vi "Get 2D String.vi"(5 "format string (%s)":string="%s", 7 "key description":string, 8 "sections":string[](array[string]), 9 "string":string[][](array[string]), 11 "info data":string) -> (0 "sections out":string[](array[string]), 2 "value":string[][](array[string]), 3 "info data out":string)   [LabVIEW 2019, in "infolib.lvlib"]
doc: "Reads matrix of strings. If section is entered it searches the key in the section(s)."
uses:
  infolib.lvlib
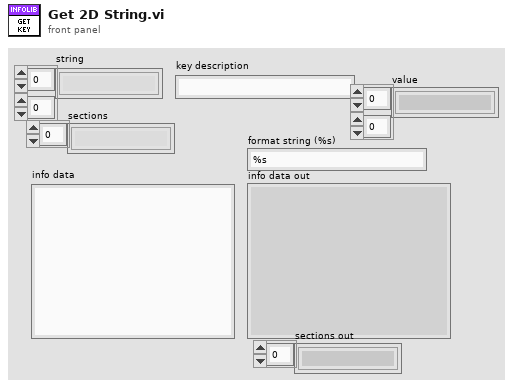
[diagram p1: front panel]
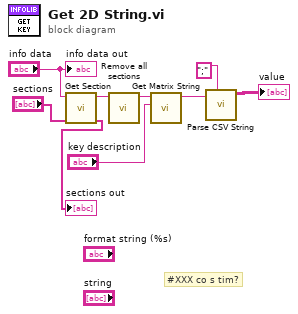
[diagram p0: block diagram]
diagram:
  # "#XXX co s tim?"
  n1 = call "Get Section.vi"("sections"="sections", "info data"="info data") -> ("sections out"=→"sections out":string[], "section part"=w9:string)  [unwired: 7 in, 1 out]
  n2 = call "Remove all sections.vi"("info data"=w9) -> ("info data out"=w7:string)  [unwired: 10 in]
  n3 = call "Get Matrix String.vi"("matrix key"="key description", "info data"=w7) -> ("matrix part"=w5:string)  [unwired: 8 in, 1 out]
  n4 = call "Parse CSV String.vi"("delimiter (,)"=";" ("delimiter (Tab)"), "CSV string"=w5) -> ("2-D array"=→"value":string[][])  [unwired: 8 in, 1 out]
  "info data out" <- "info data"
